vi "Trigger External Configure.vi"(8 "error in (no error)":errorcluster {"code" format="%.0x"}, 9 "ExternalTriggerSlope (Positive)":i32(ring)=1 items=["Positive"=1, "Negative"=2], 10 "ExternalTriggerLevel":dbl, 11 "instrument handle":refnum<k15>) -> (0 "error out":errorcluster {"code" format="%.0x"}, 3 "instrument handle out":refnum<k15>)   [LabVIEW 2009, in "Keysight XSAn.lvlib"]
doc: "This VI specifies the external level and slope for triggering.\n\nSupported Models: All supported"
uses:
  <instrlib>/Keysight XSAn/Keysight XSAn.lvlib
  AgXSAn.dll
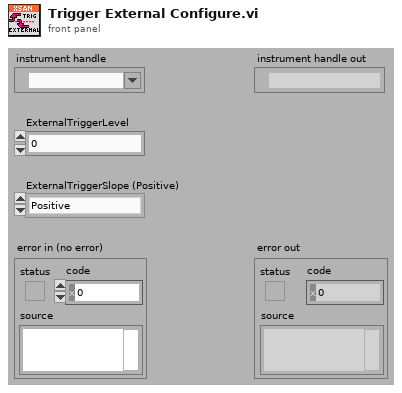
[diagram p1: front panel]
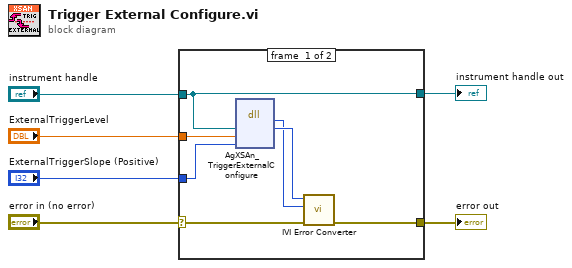
[diagram p0: block diagram]
diagram:
  n1 = case shown="No Error" "error in (no error)" {
    selector: "error in (no error)" -> [w8 w15]
    tunnel: [w9 w15] -> w6
    tunnel: "instrument handle" -> [w7 w14]
    tunnel: "ExternalTriggerLevel" -> [w13 _]
    tunnel: "ExternalTriggerSlope (Positive)" -> [w12 _]
    tunnel: [w7 w14] -> w1
    frame #0 {
      n2 = dll-call lib="AgXSAn**.dll" fn="AgXSAn_TriggerExternalConfigure"("Vi"=w7, "ExternalTriggerLevel"=w13, "ExternalTriggerSlope"=w12) -> (w10:i32, "Vi"=w11:u32)  [unwired: 5 in, 2 out]
      n3 = call <instrlib>:"IVI Error Converter.vi"("error in (no error)"=w8, "IVI error code (0)"=w10, "instrument handle"=w11) -> ("error out"=w9:errorcluster)  [unwired: 7 in, 1 out]
    }
    frame #1 {
    }
  }
  "error out" <- w6
  "instrument handle out" <- w1
